vi "Voltage Cycle.vi"() -> ()   [LabVIEW 2015]
uses:
  <instrlib>/Agilent E363X Series/Agilent E363X Series.lvlib
panel:
  out "Python Error":string
  out "Output":string
  in  "?":bool
  in  "Data Input":path
  in  "Delay Control":dbl format="%#_g seconds"
  in  "Ending Voltage":dbl format="%#_g V"
  in  "Voltage Step":dbl format="%#_g V"
  out "# Trials":dbl
  in  "BLE Serial No.":string
  in  "Starting Voltage":dbl format="%#_g V"
  in  "Current Limit (1.0 A)":dbl=1.0 format="%.3g"
  out "Actual Current Level (A)":dbl format="%.3g"
  out "Actual Voltage Level (V)":dbl format="%.3g"
  in  "VISA resource name":refnum<visa-resource-name>
  in  "start":bool
  in  "# Measurements":dbl format="%#_g "
  in  "Time inbetween Trials":dbl format="%#_g seconds"
  in  "Time inbetween Measurements":dbl format="%#_g seconds"
  out "Voltage":dbl(knob) scale=-25.0..25.0
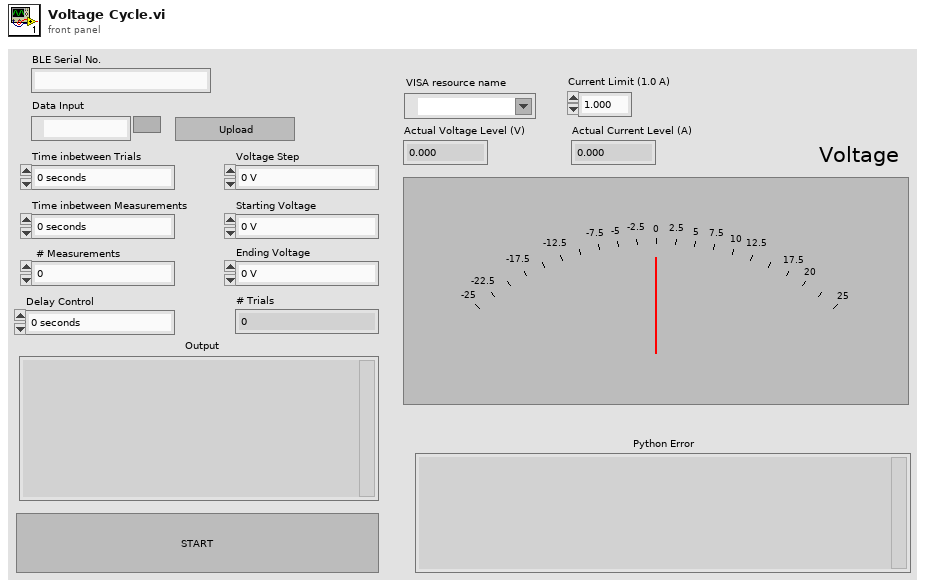
[diagram p1: front panel]
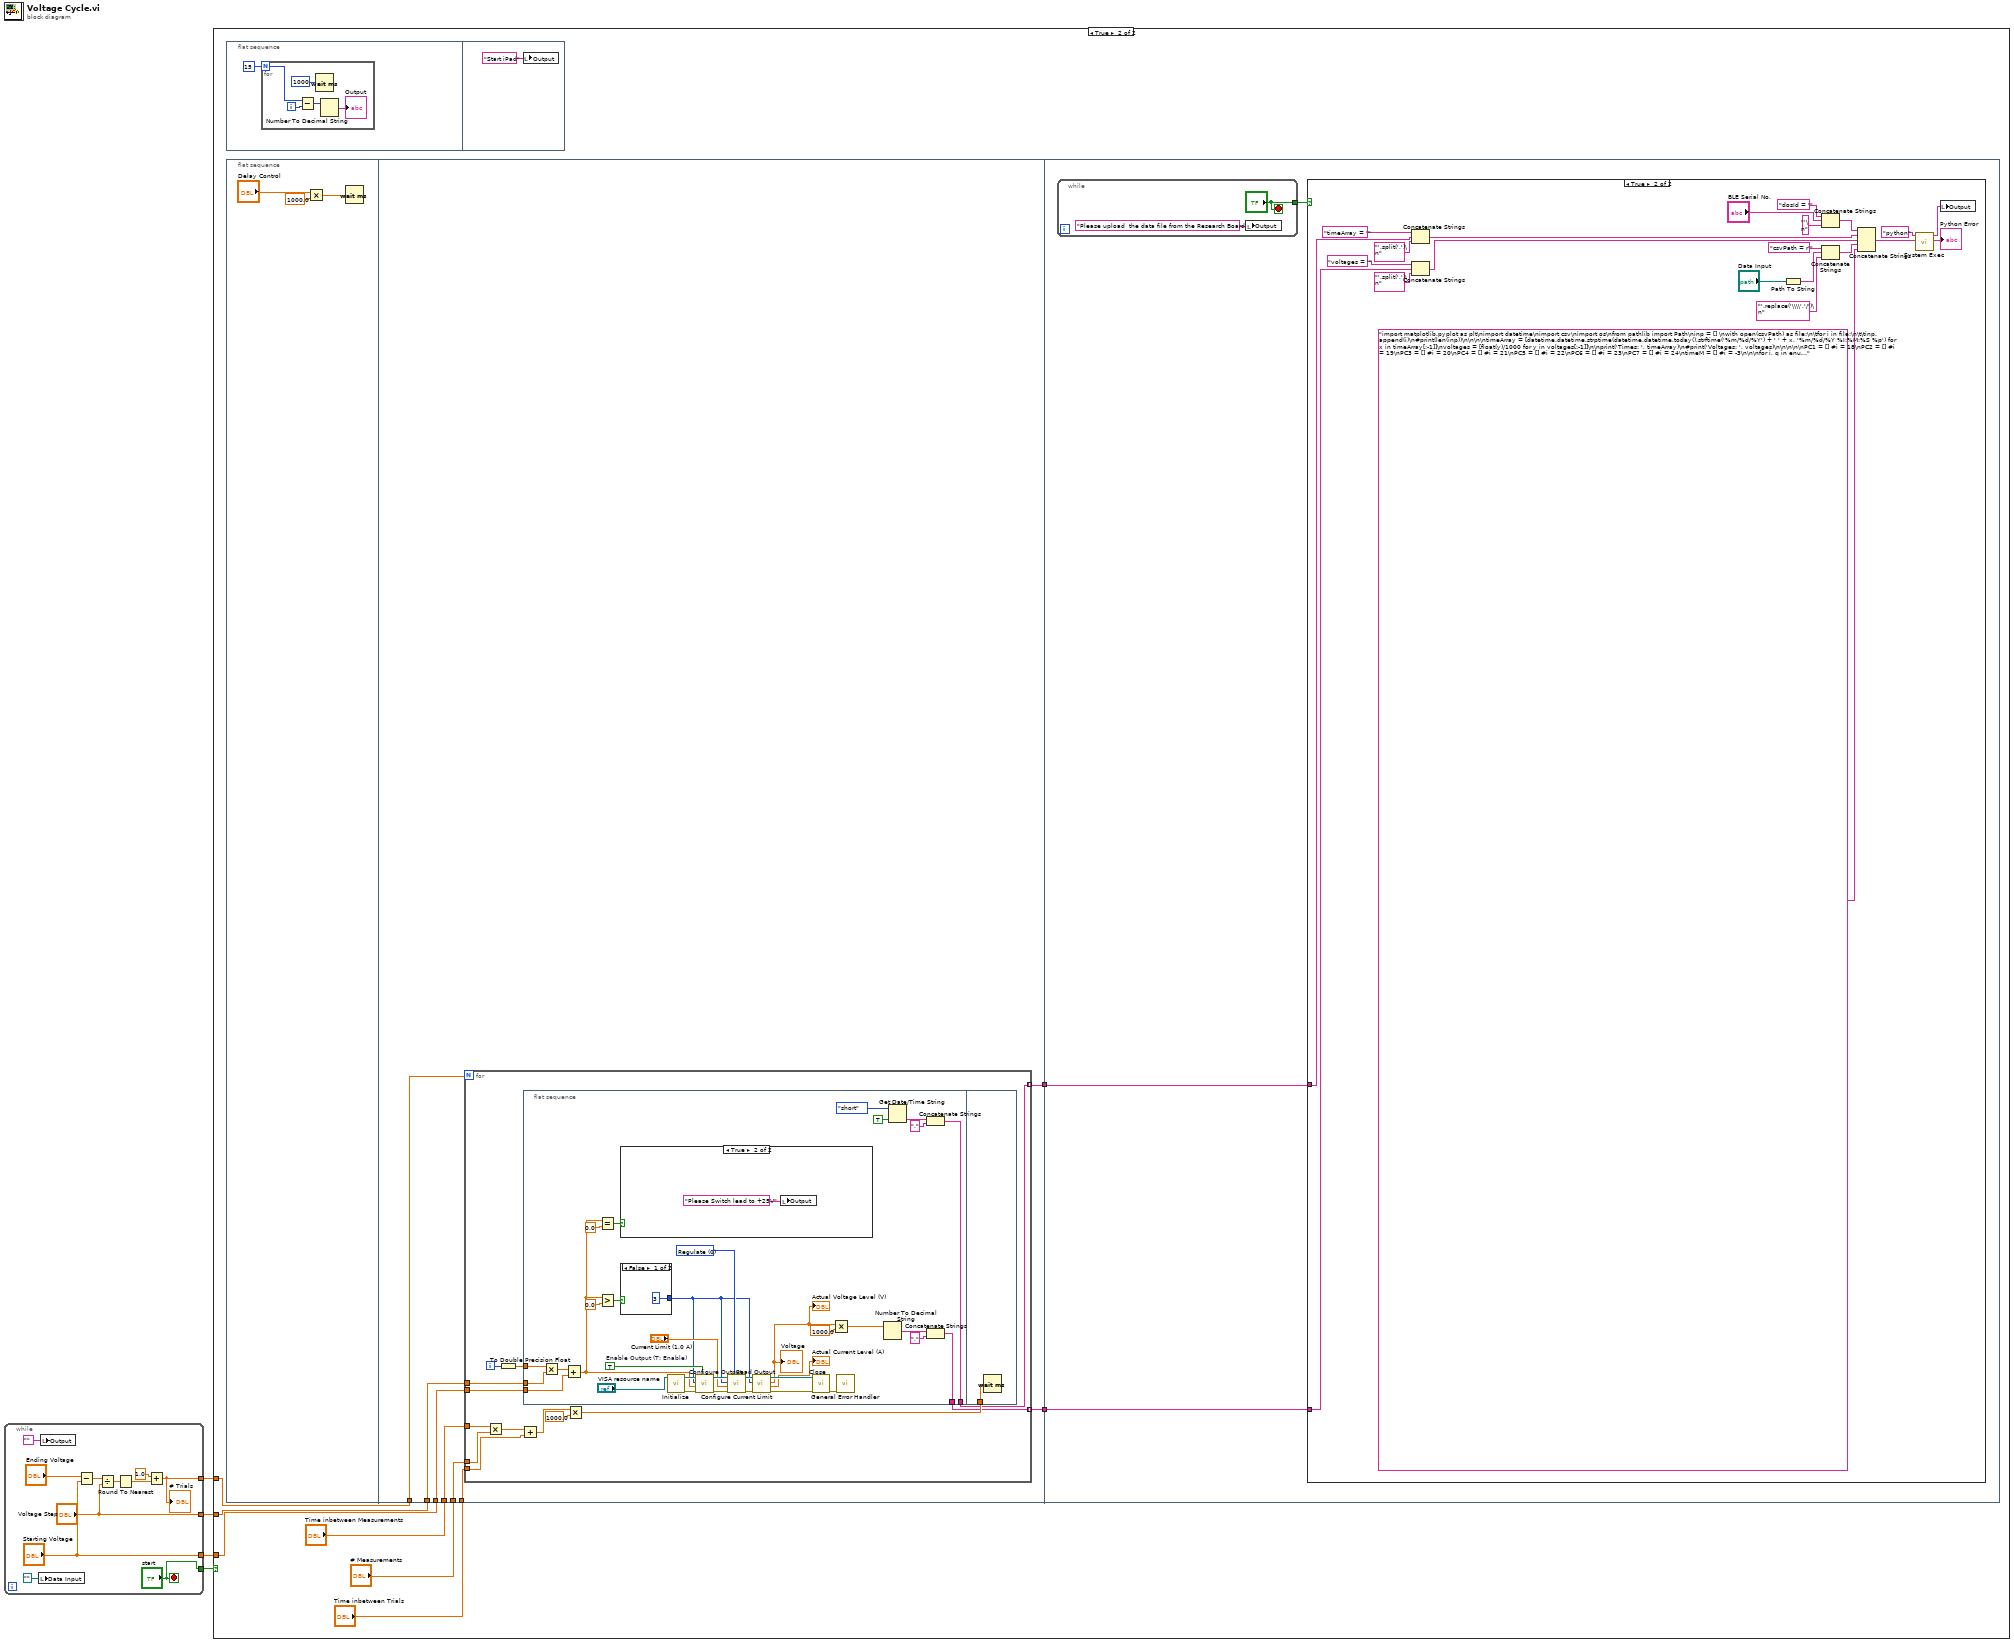
[diagram p0: block diagram]
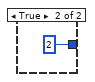
[diagram p4: hidden frame]
diagram:
  n1 = while {
    tunnel: ["start"] -> w2
    tunnel: [w11] -> w3
    tunnel: ["Voltage Step"] -> w4
    tunnel: ["Starting Voltage"] -> w1
    stop <- "start" stop-if-true
    n2 = local write "Data Input"(path "") -> ()
    n3 = local write "Output"("") -> ()
    n4 = Subtract(x="Ending Voltage", y="Starting Voltage") -> (x-y=w7:dbl)
    n5 = Divide(x=w7, y="Voltage Step") -> (x/y=w13:dbl)
    n6 = Round To Nearest(number=w13) -> (nearest integer value=w12:dbl)
    n7 = Add(x=1.0, y=w12) -> (x+y=w11:dbl)
    "# Trials" <- w11
  }
  n8 = case shown="True" w2 {
    tunnel: w3 -> [_ w22]
    tunnel: w4 -> [_ w19]
    tunnel: w1 -> [_ w16]
    frame False {
    }
    frame True {
      n9 = flat-sequence {
        frame #0 {
          n10 = for {
            N: 15 -> [w119]
            i -> [w118]
            n11 = Subtract(x=w119, y=w118) -> (x-y=w117:i32)
            n12 = Wait (ms)(milliseconds to wait=u32 1000) -> ()  [unwired: 1 out]
            n13 = Number To Decimal String(number=w117) -> (decimal integer string=→"Output":string)  [unwired: 1 in]
          }
        }
        frame #1 {
          n14 = local write "Output"("Start iPad") -> ()
        }
      }
      n15 = flat-sequence {
        tunnel: "Time inbetween Measurements" -> [w34]
        tunnel: w22 -> [w30]
        tunnel: "# Measurements" -> [w33]
        tunnel: "Time inbetween Trials" -> [w32]
        tunnel: w19 -> [w31]
        tunnel: [w29] -> w18
        tunnel: [w28] -> w17
        tunnel: w16 -> [w27]
        tunnel: w18 -> [w88]
        tunnel: w17 -> [w87]
        frame #0 {
          n16 = Multiply(x="Delay Control", y=1000.0) -> (x*y=w24:dbl)
          n17 = Wait (ms)(milliseconds to wait=w24) -> ()  [unwired: 1 out]
        }
        frame #1 {
          n18 = for {
            N: w30 -> [_]
            tunnel: w34 -> [w43]
            tunnel: w33 -> [w42]
            tunnel: w32 -> [w41]
            tunnel: w31 -> [w40]
            tunnel: [w37] -> w29 mode=indexing
            tunnel: [w36] -> w28 mode=indexing
            tunnel: w27 -> [w35]
            i -> [w38]
            n19 = Multiply(x=w43, y=w42) -> (x*y=w47:dbl)
            n20 = To Double Precision Float(number=w38) -> (double precision float=w39:dbl)
            n21 = Add(x=w47, y=w41) -> (x+y=w46:dbl)
            n22 = flat-sequence {
              tunnel: w40 -> [w62]
              tunnel: w39 -> [w61]
              tunnel: [w58] -> w37
              tunnel: [w55] -> w36
              tunnel: w35 -> [w54]
              tunnel: w44 -> [w86]
              frame #0 {
                w69 = u16 0 items=["Regulate", "Trip"] ("Behavior (0: Regulate)")
                w78 = TRUE  # Enable Output (T: Enable)
                n23 = Multiply(x=w61, y=w62) -> (x*y=w68:dbl)
                n24 = Add(x=w68, y=w54) -> (x+y=w49:dbl)
                n25 = Equal?(x=w49, y=0.0) -> (x = y?=w48:bool)
                n26 = Greater?(x=w49, y=0.0) -> (0:w52:bool)
                n27 = case shown="True" w48 {
                  frame False {
                  }
                  frame True {
                    n28 = local write "Output"("Please Switch lead to +25V") -> ()
                  }
                }
                n29 = case shown="False" w52 {
                  tunnel: [3 2] -> w51
                  frame False {
                  }
                  frame True {
                  }
                }
                n30 = call <instrlib>:"Initialize.vi"("VISA resource name"="VISA resource name") -> ("error out"=w79:errorcluster, "VISA resource name out"=w81:refnum<visa-resource-name>)  [unwired: 9 in]
                n31 = call <instrlib>:"Configure Output.vi"("Enable Output (T: Enable)"=w78, "error in (no error)"=w79, "Voltage Level (0.0 V)"=w49, "Channel (1: Channel 1)"=w51, "VISA resource name"=w81) -> ("error out"=w73:errorcluster, "VISA resource name out"=w74:refnum<visa-resource-name>)  [unwired: 5 in]
                n32 = call <instrlib>:"Configure Current Limit.vi"("Behavior (0: Regulate)"=w69, "error in (no error)"=w73, "Current Limit (0.0 A)"="Current Limit (1.0 A)", "Channel (1: Channel 1)"=w51, "VISA resource name"=w74) -> ("error out"=w72:errorcluster, "VISA resource name out"=w71:refnum<visa-resource-name>)  [unwired: 5 in]
                n33 = call <instrlib>:"Read Output.vi"("error in (no error)"=w72, "Channel (1: Channel 1)"=w51, "VISA resource name"=w71) -> ("error out"=w77:errorcluster, "Actual Current Level (A)"=→"Actual Current Level (A)":dbl, "Actual Voltage Level (V)"=w65:dbl, "VISA resource name out"=w76:refnum<visa-resource-name>)  [unwired: 5 in]
                "Voltage" <- w65
                "Actual Voltage Level (V)" <- w65
                n34 = call <instrlib>:"Close.vi"("error in (no error)"=w77, "VISA resource name"=w76) -> ("error out"=w80:errorcluster)  [unwired: 9 in]
                n35 = Multiply(x=w65, y=1000.0) -> (x*y=w63:dbl)
                n36 = call <vilib>:"General Error Handler.vi"("error in (no error)"=w80) -> ()  [unwired: 10 in, 5 out]
                n37 = Number To Decimal String(number=w63) -> (decimal integer string=w57:string)  [unwired: 1 in]
                n38 = Get Date/Time String(date format (0)=enum16{"short", "long", "abbreviated"}."short", want seconds? (F)=TRUE) -> (time string=w60:string)  [unwired: 1 in, 1 out]
                n39 = Concatenate Strings(w60, ",") -> (w58:string)
                n40 = Concatenate Strings(w57, ",") -> (w55:string)
              }
              frame #1 {
                n41 = Wait (ms)(milliseconds to wait=w86) -> ()  [unwired: 1 out]
              }
            }
            n42 = Multiply(x=w46, y=1000.0 ("x")) -> (x*y=w44:dbl)
          }
        }
        frame #2 {
          n43 = while {
            tunnel: ["?"] -> w89
            stop <- "?" stop-if-true
            n44 = local write "Output"("Please upload  the data file from the Research Board") -> ()
          }
          n45 = case shown="True" w89 {
            tunnel: w88 -> [_ w92]
            tunnel: w87 -> [_ w91]
            frame False {
            }
            frame True {
              n46 = Concatenate Strings("timeArray = '", w92, "'.split(',')\n") -> (w105:string)
              n47 = Concatenate Strings("voltages = '", w91, "'.split(',')\n") -> (w106:string)
              n48 = Path To String(path="Data Input") -> (string=w93:string)
              n49 = Concatenate Strings("dosId = '", "BLE Serial No.", "'\n") -> (w104:string)
              n50 = Concatenate Strings("csvPath = r'", w93, "'.replace('\\\\','/')\n") -> (w107:string)
              n51 = Concatenate Strings(w104, w105, w106, w107, "import matplotlib.pyplot as plt\nimport datetime\nimport csv\nimport os\nfrom pathlib import Path\ninp = [] \nwith open(csvPath) as file:\n\tfor i in file:\n\t\tinp.append(i)\n#print(len(inp))\n\n\n\ntimeArray = [datetime.datetime.strptime(datetime.datetime.today().strftime('%m/%d/%Y') + ' ' + x, '%m/%d/%Y %I:%M:%S %p') for x in timeArray[:-1]]\nvoltages = [float(y)/1000 for y in voltages[:-1]]\n\nprint('Times: ', timeArray)\n#print('Voltages: ', voltages)\n\n\n\n\nPC1 = [] #i = 18\nPC2 = [] #i = 19\nPC3 = [] #i = 20\nPC4 = [] #i = 21\nPC5 = [] #i = 22\nPC6 = [] #i = 23\nPC7 = [] #i = 24\ntimeM = [] #i = -3\n\n\nfor i, q in enumerate(inp):\n       # print(i, q)\n        if i > 1:\n                data = q.split(',')\n                if data[6] == dosId:\n                        PC1.append(float(data[18]))\n                        PC2.append(float(data[19]))\n                        PC3.append(float(data[20]))\n                        PC4.append(float(data[21]))\n                        PC5.append(float(data[22]))\n                        PC6.append(float(data[23]))\n                        PC7.append(float(data[24]))\n                        timeM.append(datetime.datetime.fromtimestamp(float(data[-3])))\n\nfullData = [PC1, PC2, PC3, PC4, PC5, PC6, PC7]\n#for q,i in enumerate(fullData):\n#        print(\"PC{0}\".format(q+1))\n#        print(i)\n\nprint(timeM)\npc1ByVolt = []\npc2ByVolt = []\npc3ByVolt = []\npc4ByVolt = []\npc5ByVolt = []\npc6ByVolt = []\npc7ByVolt = []\n\nfor ind, vTime in enumerate(timeArray):\n        volt1 = []\n        volt2 = []\n        volt3 = []\n        volt4 = []\n        volt5 = []\n        volt6 = []\n        volt7 = []\n        zeit = timeM[ind]\n\n        print(\"Time from LV: {0} Time from Data: {1}\".format(vTime, zeit))\n        \n        if vTime < zeit:\n                if ind + 1 < len(timeArray):\n                        if zeit < timeArray[ind+1]:\n                                print(\"Successfully appended data from index {0}\".format(ind))\n                                volt1.append(PC1[ind])\n                                volt2.append(PC2[ind])\n                                volt3.append(PC3[ind])\n                                volt4.append(PC4[ind])\n                                volt5.append(PC5[ind])\n                                volt6.append(PC6[ind])\n                                volt7.append(PC7[ind])\n                else :\n                        print(\"No further time\")\n                        volt1.append(PC1[ind])\n                        volt2.append(PC2[ind])\n                        volt3.append(PC3[ind])\n                        volt4.append(PC4[ind])\n                        volt5.append(PC5[ind])\n                        volt6.append(PC6[ind])\n                        volt7.append(PC7[ind]) \n        pc1ByVolt.append(volt1)\n        pc2ByVolt.append(volt2)\n        pc3ByVolt.append(volt3)\n        pc4ByVolt.append(volt4)\n        pc5ByVolt.append(volt5)\n        pc6ByVolt.append(volt6)\n        pc7ByVolt.append(volt7)\n\nallDataByVolt = [pc1ByVolt, pc2ByVolt, pc3ByVolt, pc4ByVolt, pc5ByVolt, pc6ByVolt, pc7ByVolt]\nfor debug in allDataByVolt:\n        print(debug)\n\nallData = []\nfor pc in allDataByVolt:\n        newPC = []\n        for volt in pc:\n                newPC.append(sum(volt)/len(volt))\n        allData.append(newPC)\n\n\nprint(allData)\nprint(allData[0])\n\nwith open(os.path.expanduser('~') + \"/Desktop/CVOutput\" + datetime.datetime.now().strftime('%I%M%S') + '.csv', 'w', newline='') as csvOut:\n        writer = csv.writer(csvOut)\n        writer.writerow([\"Measurement Time\", \"Voltage\", \"PC1\", \"PC2\", \"PC3\", \"PC4\", \"PC5\", \"PC6\", \"PC7\"])\n        for i, time in enumerate(timeM):\n                print(i)\n                writer.writerow([time, voltages[i], allData[0][i], allData[1][i], allData[2][i], allData[3][i], allData[4][i], allData[5][i], allData[6][i]])\n\nfor pc, i in enumerate(allData):\n        plt.figure(pc+1)\n        plt.plot(voltages, i)\n        plt.xlabel(\"Voltage (V)\")\n        plt.ylabel(\"Capacitance (fF)\")\n        plt.title(\"PC{0}\".format(pc+1) + \" Inf: NaN\")\n        plt.grid(True)\nplt.show(block=True)\n") -> (w90:string)
              n52 = call <vilib>:"System Exec.vi"("standard input"=w90, "command line"="python") -> ("standard error"=→"Python Error":string, "standard output"=w110:string)  [unwired: 6 in, 2 out]
              n53 = local write "Output"(w110) -> ()
            }
          }
        }
      }
    }
  }
